vi "bmp085_get_up.vi"(8 "error in (no error)":errorcluster, 11 "BMP085 (GY-65) in":refnum<class "BMP085 (GY-65).lvclass">) -> (0 "error out":errorcluster, 2 "UP":i32, 3 "BMP085 (GY-65) out":refnum<class "BMP085 (GY-65).lvclass">)   [LabVIEW 2015, in "BMP085 (RT).lvlib" / "BMP085 (GY-65).lvclass"]
uses:
  BMP085 (GY-65).lvclass
  BMP085 (GY-65).lvclass/BMP085 (GY-65).ctl
  <vilib>/Utility/error.llb/Error Cluster From Error Code.vi
  <vilib>/myRIO/Common/Instrument Driver Framework/myRIO v1.0/I2C/vis/myRIO v1.0 Write I2C.vi
  <vilib>/myRIO/Common/Instrument Driver Framework/myRIO v1.0/I2C/vis/myRIO v1.0 Read I2C.vi
  <vilib>/myRIO/Instrument Drivers/Onboard IO/I2C/I2C.lvlib
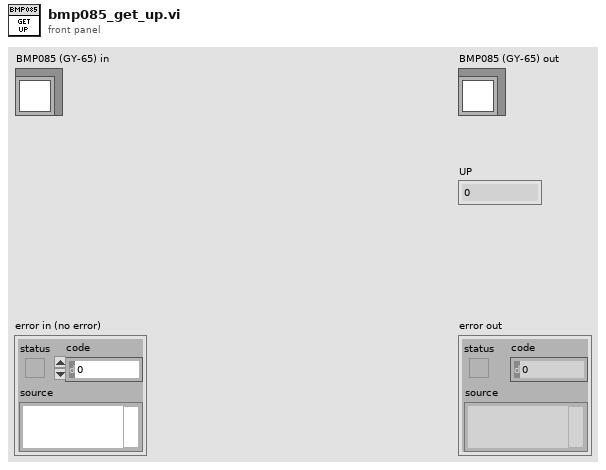
[diagram p1: front panel]
types:
  T1 = typedef "I2C.lvlib/I2C Reference.ctl" = cluster{"myRIO Reference":T2, "I2C Channels Enum":T6, "I2C Configuration":T7}
  T2 = typedef "myRIO Generic Hardware Reference.ctl" = cluster{"myRIO Model":T3, "myRIO Hardware Reference":T4}
  T3 = typedef "Hardware Version Enum.ctl" = enum16{"Unknown", "myRIO-1900", "myRIO-1950", "roboRIO"}
  T4 = typedef "myRIO v1.0 Reference.ctl" = cluster{"Generic FPGA Reference":T5, "Allow multiple opens":bool}
  T5 = typedef "Generic FPGA Reference.ctl" = refnum<k20>
  T6 = typedef "I2C Channels Enum.ctl" = enum16{"Not Connected", "A/I2C", "B/I2C", "I2C/I2C"}
  T7 = typedef "I2C.lvlib/I2C Configuration.ctl" = cluster{"I2C Transfer Rate":T8}
  T8 = typedef "I2C.lvlib/I2C Transfer Rate.ctl" = enum16{"Standard mode (100 kbps)", "Fast mode (400 kbps)"}
  T9 = enum8{"ultra low power", "standard", "high resolution", "ultra high resolution"}
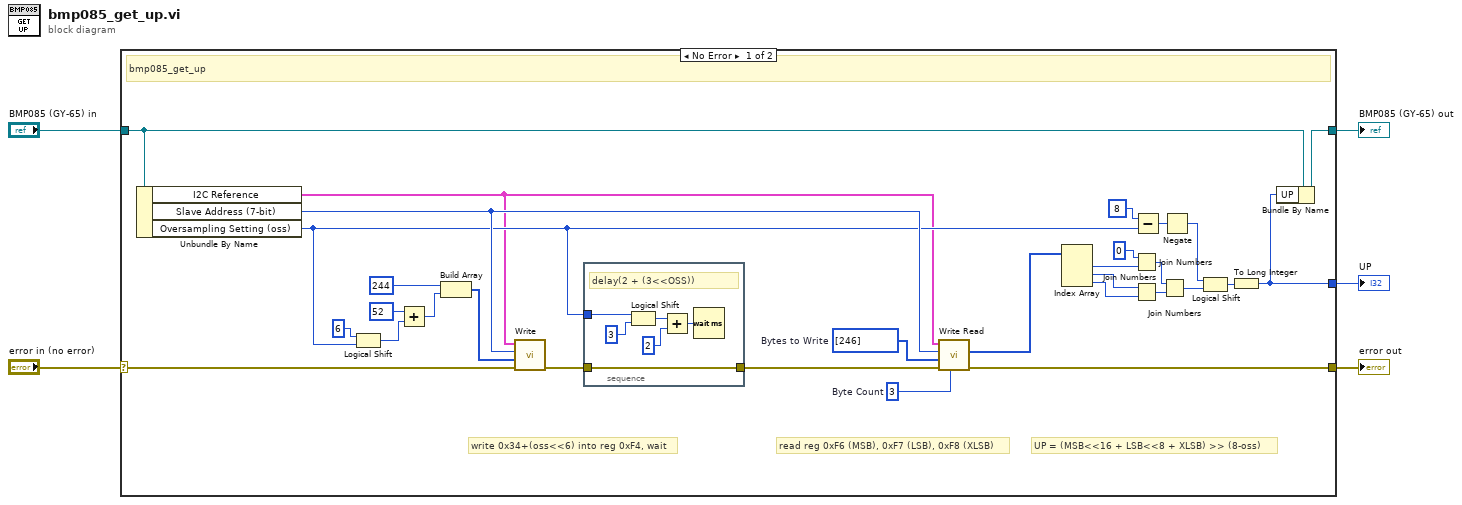
[diagram p0: block diagram]
diagram:
  n1 = case shown="No Error" "error in (no error)" {
    selector: "error in (no error)" -> [w34 w43]
    tunnel: [w9 w43] -> w4
    tunnel: [w8 w42] -> w2
    tunnel: "BMP085 (GY-65) in" -> [w35 w42]
    tunnel: [w6 _] -> w1
    frame No Error {
      w25 = u32 3  # Byte Count
      w24 = u8[] [246]  # Bytes to Write
      # "read reg 0xF6 (MSB), 0xF7 (LSB), 0xF8 (XLSB)"
      # "write 0x34+(oss<<6) into reg 0xF4, wait"
      # "UP = (MSB<<16 + LSB<<8 + XLSB) >> (8-oss)"
      # "bmp085_get_up"
      n2 = Unbundle By Name(w35) -> ("I2C Reference"=w7:T1, "Slave Address (7-bit)"=w23:u8, "Oversampling Setting (oss)"=w10:T9)
      n3 = Logical Shift(y=u8 6, x=w10) -> (x << y=w28:u32)
      n4 = Add(x=u8 52, y=w28) -> (x+y=w29:u8)
      n5 = Build Array(u8 244, w29) -> (w30:u8[])
      n6 = call <vilib>:"Write.vi"("error in (no error)"=w34, "Bytes to Write"=w30, "Slave Address (7-bit)"=w23, "I2C Ref In"=w7) -> ("error out"=w27:errorcluster)  [unwired: 6 in, 1 out]
      n7 = stacked-sequence {
        tunnel: w27 -> [w41]
        tunnel: [w41] -> w26
        tunnel: w10 -> [w36]
        frame #0 {
          # "delay(2 + (3<<OSS))"
          n8 = Logical Shift(y=w36, x=u8 3) -> (x << y=w39:u8)
          n9 = Add(x=w39, y=2) -> (x+y=w37:u32)
          n10 = Wait (ms)(milliseconds to wait=w37) -> ()  [unwired: 1 out]
        }
      }
      n11 = call <vilib>:"Write Read.vi"("Byte Count"=w25, "error in (no error)"=w26, "Bytes to Write"=w24, "Slave Address (7-bit)"=w23, "I2C Ref In"=w7) -> ("error out"=w9:errorcluster, "Bytes Read"=w11:u8[])  [unwired: 3 in, 1 out]
      n12 = Index Array(array=w11) -> (element #1=w19:u8, element #2=w20:u8, element #3=w21:u8)  [unwired: 3 in]
      n13 = Join Numbers(hi=u8 0, lo=w19) -> ((hi.lo)=w15:u16)
      n14 = Join Numbers(hi=w20, lo=w21) -> ((hi.lo)=w14:u16)
      n15 = Subtract(x=u8 8, y=w10) -> (x-y=w16:i8)
      n16 = Join Numbers(hi=w15, lo=w14) -> ((hi.lo)=w22:u32)
      n17 = Negate(x=w16) -> (-x=w17:i8)
      n18 = Logical Shift(y=w17, x=w22) -> (x << y=w18:u32)
      n19 = To Long Integer(number=w18) -> (32bit integer=w6:i32)
      n20 = Bundle By Name(cluster=w35, "UP"=w6) -> (w8:refnum<class "BMP085 (GY-65).lvclass">)
    }
    frame Error {
    }
  }
  "error out" <- w4
  "BMP085 (GY-65) out" <- w2
  "UP" <- w1
